vi "Setra Data Parse.vi"(8 "Error In":errorcluster, 10 "Input Data":string=" -17.804  PS\r\n") -> (0 "Error Out":errorcluster, 2 "Output Data":string=" -17.804  PS\r\n", 4 "Data & Stability":bool, 6 "Weight":dbl)   [LabVIEW 2016]
uses:
  <vilib>/Utility/error.llb/whitespace.ctl
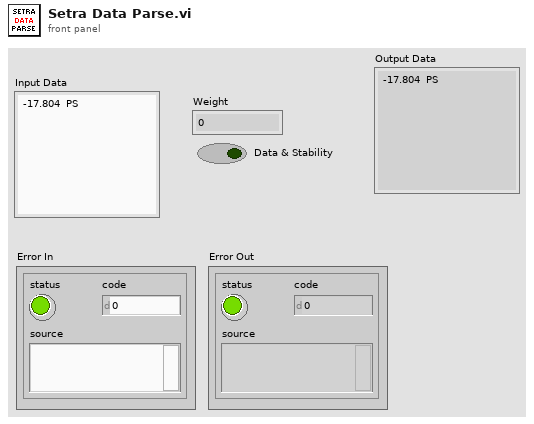
[diagram p1: front panel]
types:
  T1 = typedef "whitespace.ctl" = u16
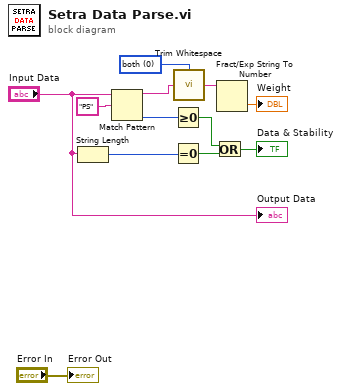
[diagram p0: block diagram]
diagram:
  w3 = T1 0 items=["both", "start of string", "end of string"] ("location (both)")
  n1 = String Length(string="Input Data") -> (length=w11:i32)
  n2 = Match Pattern(string="Input Data", regular expression="PS") -> (before substring=w4:string, offset past match=w8:i32)  [unwired: 1 in, 2 out]
  n3 = Greater Or Equal To 0?(x=w8) -> (x >= 0?=w9:bool)
  n4 = Equal To 0?(x=w11) -> (x = 0?=w12:bool)
  n5 = call <vilib>:"Trim Whitespace.vi"("string"=w4, "location (both)"=w3) -> ("trimmed string"=w2:string)
  n6 = Or(x=w9, y=w12) -> (x .or. y?=→"Data & Stability":bool)
  n7 = Fract/Exp String To Number(string=w2) -> (number=→"Weight":dbl)  [unwired: 3 in, 1 out]
  "Error Out" <- "Error In"
  "Output Data" <- "Input Data"
